vi "Status Reg A.vi"(1 "Status:Register:A":i16) -> (0 "Reg A":i16[](array[numeric]))   [LabVIEW 2019, in "DeltaPSControl Engine.lvlib"]
uses:
  DeltaPSControl Engine.lvlib
panel:
  out "DCFV":bool
  out "Vlim":bool
  out "Ilim":bool
  out "CV":bool
  out "CC":bool
  out "FRONTPANELLOCK":bool
  out "INTERLOCK":bool
  out "RSD":bool
  out "ACF":bool
  out "OUTPUT":bool
  out "OT":bool
  out "PSOL":bool
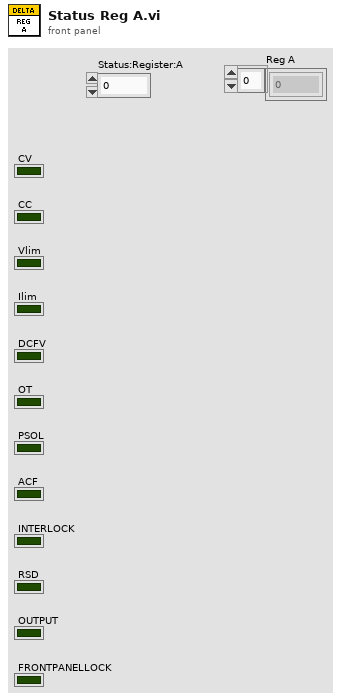
[diagram p1: front panel]
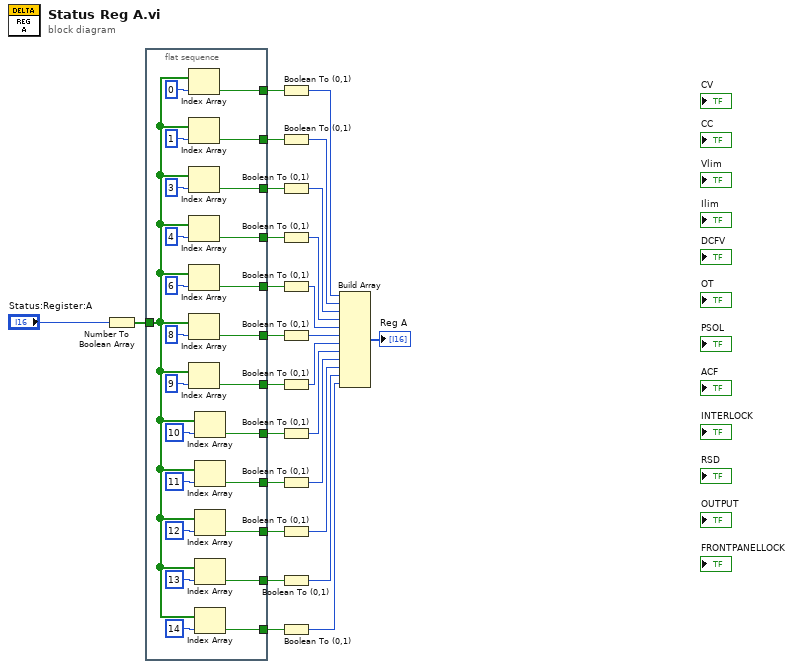
[diagram p0: block diagram]
diagram:
  n1 = Number To Boolean Array(number="Status:Register:A") -> (Boolean array=w27:bool[])
  n2 = flat-sequence {
    tunnel: [w52] -> w19
    tunnel: [w49] -> w18
    tunnel: [w44] -> w17
    tunnel: [w43] -> w16
    tunnel: [w42] -> w14
    tunnel: [w41] -> w15
    tunnel: [w39] -> w24
    tunnel: w27 -> [w33]
    tunnel: [w32] -> w25
    tunnel: [w31] -> w23
    tunnel: [w30] -> w22
    tunnel: [w29] -> w21
    tunnel: [w28] -> w20
    frame #0 {
      n3 = Index Array(array=w33, index=0) -> (element=w32:bool)
      n4 = Index Array(array=w33, index=1) -> (element=w31:bool)
      n5 = Index Array(array=w33, index=3) -> (element=w30:bool)
      n6 = Index Array(array=w33, index=4) -> (element=w29:bool)
      n7 = Index Array(array=w33, index=6) -> (element=w28:bool)
      n8 = Index Array(array=w33, index=8) -> (element=w52:bool)
      n9 = Index Array(array=w33, index=9) -> (element=w49:bool)
      n10 = Index Array(array=w33, index=10) -> (element=w44:bool)
      n11 = Index Array(array=w33, index=11) -> (element=w43:bool)
      n12 = Index Array(array=w33, index=12) -> (element=w41:bool)
      n13 = Index Array(array=w33, index=13) -> (element=w42:bool)
      n14 = Index Array(array=w33, index=14) -> (element=w39:bool)
    }
  }
  n15 = Boolean To (0,1)(Boolean=w25) -> (0, 1=w13:i16)
  n16 = Boolean To (0,1)(Boolean=w23) -> (0, 1=w12:i16)
  n17 = Boolean To (0,1)(Boolean=w22) -> (0, 1=w11:i16)
  n18 = Boolean To (0,1)(Boolean=w21) -> (0, 1=w10:i16)
  n19 = Boolean To (0,1)(Boolean=w20) -> (0, 1=w9:i16)
  n20 = Boolean To (0,1)(Boolean=w19) -> (0, 1=w8:i16)
  n21 = Boolean To (0,1)(Boolean=w18) -> (0, 1=w7:i16)
  n22 = Boolean To (0,1)(Boolean=w17) -> (0, 1=w6:i16)
  n23 = Boolean To (0,1)(Boolean=w16) -> (0, 1=w5:i16)
  n24 = Boolean To (0,1)(Boolean=w15) -> (0, 1=w4:i16)
  n25 = Boolean To (0,1)(Boolean=w14) -> (0, 1=w3:i16)
  n26 = Boolean To (0,1)(Boolean=w24) -> (0, 1=w2:i16)
  n27 = Build Array(w13, w12, w11, w10, w9, w8, w7, w6, w5, w4, w3, w2) -> (→"Reg A":i16[])
